vi "build.stepElement.parse.vi"(11 "steps in":variant[](array[variant])) -> (0 "error out":errorcluster, 3 "Flow Elements":T1[](array[typedef]))   [LabVIEW 2024]
uses:
  controls/UiStepBuilder.ctl
  controls/type.step-builder.ctl
  controls/typeStepVarients.ctl
  controls/type.StepFunction.ctl
  Polymorphics/variantCtrlString.vi
  Polymorphics/variantCtrlStepFunction.vi
  Polymorphics/variantCtrlSetpoint.vi
  Polymorphics/variantCtrlNumber.vi
  proc.util.validateParamExist.vi
  <vilib>/Utility/error.llb/Clear Errors.vi
  <vilib>/Utility/error.llb/Trim Whitespace One-Sided.vi
  util.error.create.vi
  Polymorphics/variantCtrlStepPointer.vi
  Polymorphics/variantCtrlStepProcPointer.vi
  Polymorphics/variantCtrlStepUserMessage.vi
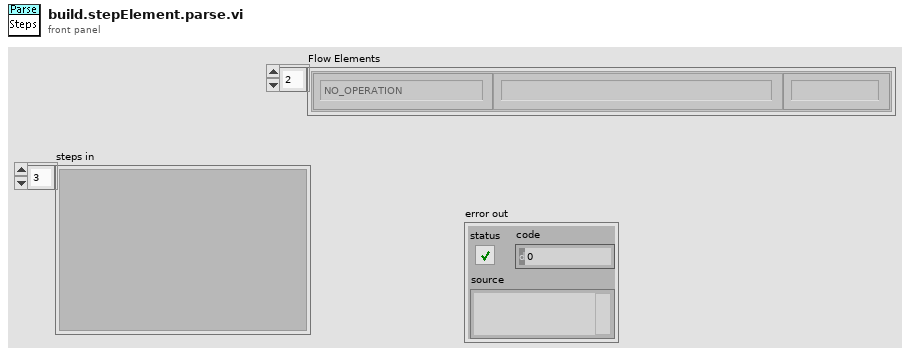
[diagram p1: front panel]
types:
  T1 = typedef "UiStepBuilder.ctl" = cluster{"Step Function":T2, "ParamString":string, "Step Label":string}
  T2 = typedef "type.step-builder.ctl" = enum16{"NO_OPERATION", "DELAY-JUMP", "DELAY", "JUMP", "COMPLETE", "SCHEDULER", "IRR-CHECK", "UNIT-CHECK", "UNIT-SAMPLE", "UNIT-DOSE", "LOG-REPORT", "LOG-MESSAGE", "IO-READ", "IO-READ-MANY", "IO-WRITE", "IO-COMPARE-OUT", "IO-COMPARE-IN", "PROC-START", "PROC-STOP", "PROC-LOAD", "PROC-IS-COMPLETED", "RECORD-MOVE", "GET-RH", "GET-UV", "GET-WD", "GET-WS", "OCS-CHECK", "OCS-RECORD"}
  T3 = typedef "typeStepVarients.ctl" = enum16{"stepNameID", "stepFunction", "stepReport", "stepSetpoint", "stepPointer", "stepProcPointer", "stepIoPointer", "stepIoValue", "stepFilePointer", "stepMessage", "stepTimeString", "stepNumReg", "stepStrReg", "stepSeconds", "stepUnitDoseParams", "stepUnitIndex"}
  T4 = typedef "type.StepFunction.ctl" = enum16{"__NO-OP", "_DELAY_LOAD", "_DELAY_COMPARE", "_JUMP", "_COMPLETE", "_COMPARE", "_LOG_MESSAGE", "_LOG_LAST_REPORT", "_SCHEDULE", "_SCHED_DAILY", "CLK_COMPARE", "PROC_START", "PROC_STOP", "PROC_LOAD", "PROC_COMPLETION_CHECK", "PROC_COMPLETION_LOAD", "_IO_READ", "_IO_READ_MANY", "_IO_WRITE", "_IO_WRITE_BY_REG", "_IO_GET_OUTPUT", "_OCS_CHECK", "_OCS_RECORD", "_GET_RH", "_GET_ACC_UV", "_GET_WD", "_GET_WS", "_REC_DELETE", "_REC_MOVE", "_REC_COPY", "_IRR_CHECK", "UNIT_CHECK", "UNIT_SAMPLE", "UNIT_DOSE"}
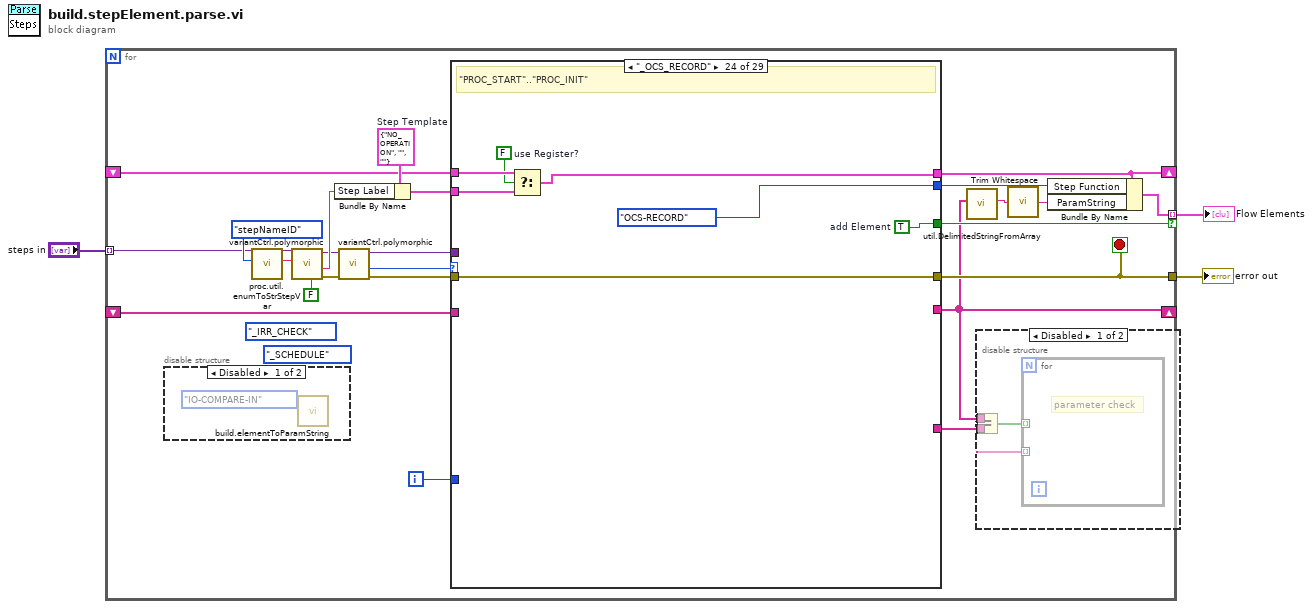
[diagram p0: block diagram]
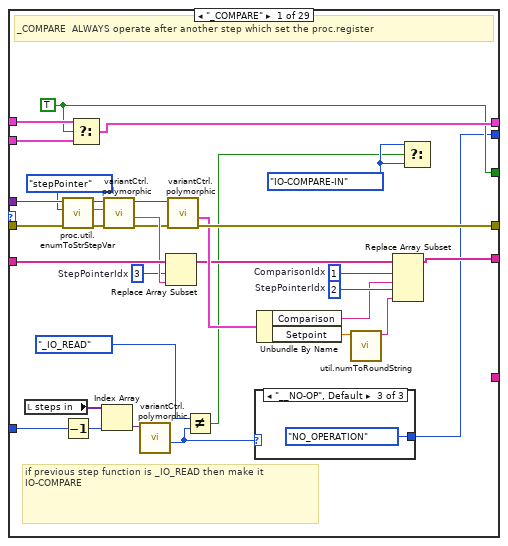
[diagram p4: hidden frame]
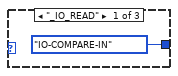
[diagram p5: hidden frame]
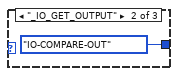
[diagram p6: hidden frame]
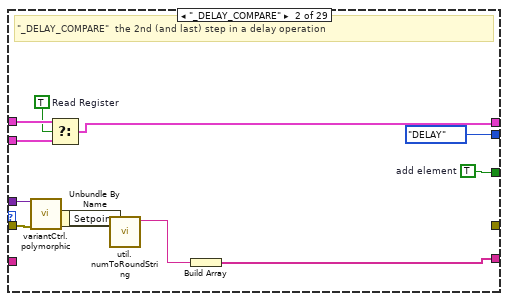
[diagram p7: hidden frame]
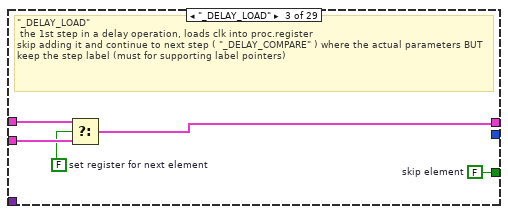
[diagram p8: hidden frame]
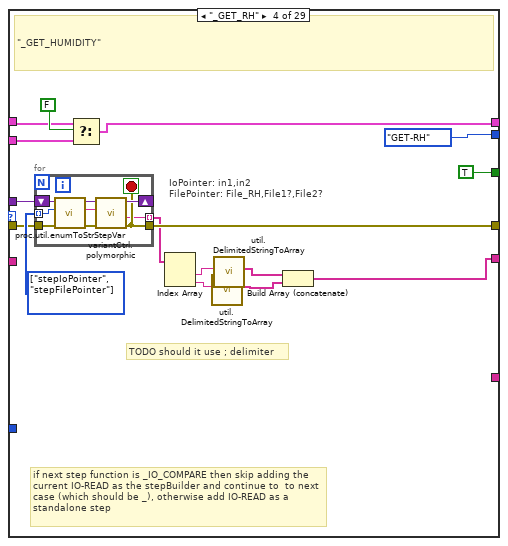
[diagram p9: hidden frame]
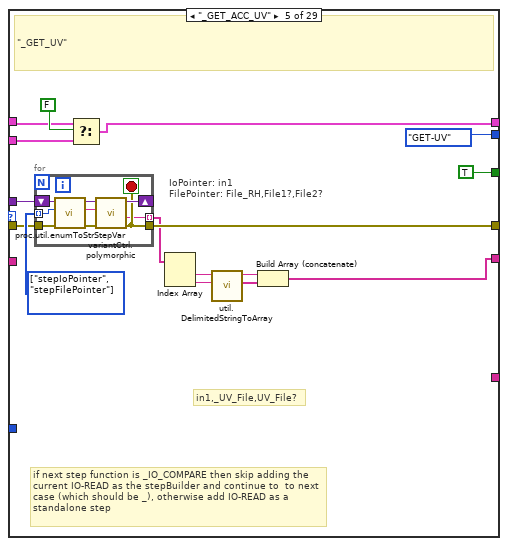
[diagram p10: hidden frame]
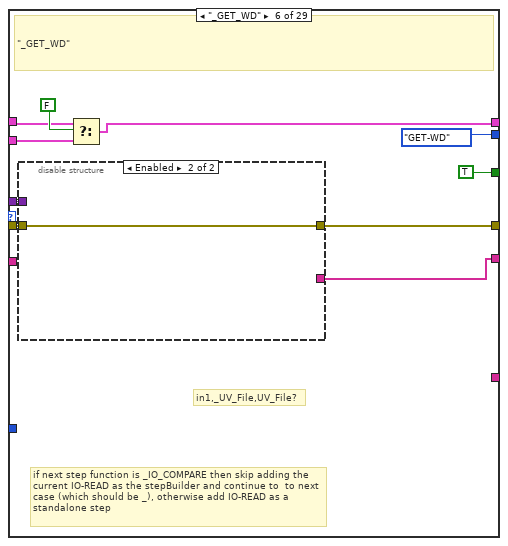
[diagram p11: hidden frame]
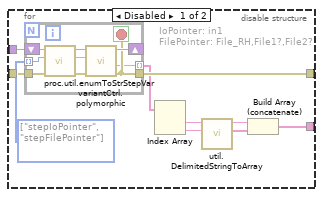
[diagram p12: hidden frame]
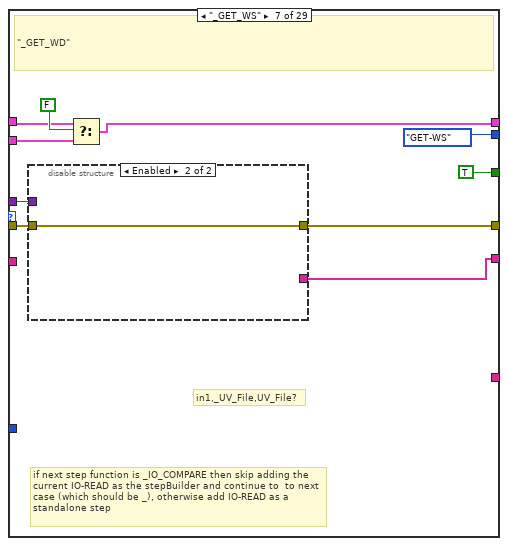
[diagram p13: hidden frame]
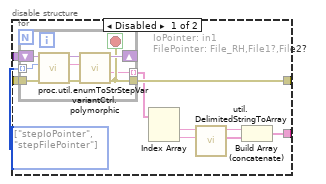
[diagram p14: hidden frame]
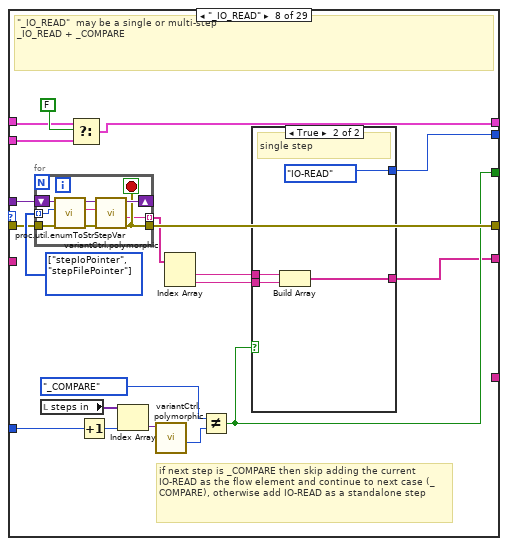
[diagram p15: hidden frame]
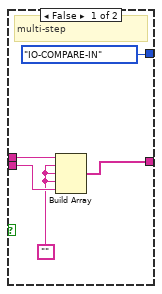
[diagram p16: hidden frame]
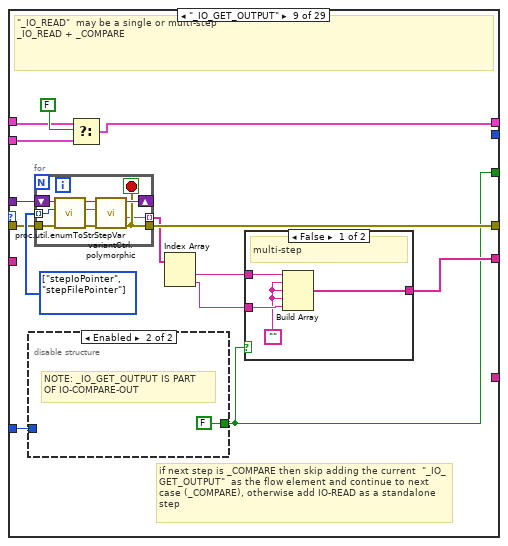
[diagram p17: hidden frame]
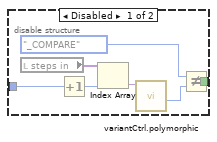
[diagram p18: hidden frame]
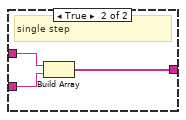
[diagram p19: hidden frame]
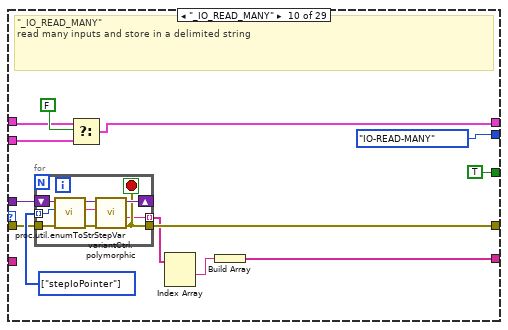
[diagram p20: hidden frame]
diagram:
  n1 = for {
    tunnel: "steps in" -> [w25] mode=indexing
    shift-right: [w9] -> _
    shift-left: _ -> [w18]
    tunnel: [w15] -> w2
    tunnel: [w10] -> w3 mode=indexing if=w14
    shift-right: [w5] -> _
    shift-left: _ -> [w13]
    i -> [w12]
    stop <- w15 stop-if-true
    (unwired) type.StepFunction."_SCHEDULE" ("StepFunction")
    (unwired) type.StepFunction."_IRR_CHECK" ("StepFunction")
    w22 = T1 {"Step Function"=enum."NO_OPERATION", "ParamString"="", "Step Label"=""}  # Step Template
    n2 = disable-structure shown="Disabled" {
      frame Disabled {
        n3 = call "build.elementToParamString.vi"("UiStepFunction"=type.step-builder."IO-COMPARE-IN") -> ()  [unwired: 9 in, 2 out]
      }
      frame Enabled {
      }
    }
    n4 = call "proc.util.enumToStrStepVar.vi"("Step var"=typeStepVarients."stepNameID") -> ("String"=w27:string)  [unwired: 10 in]
    n5 = call-poly "variantCtrl.polymorphic.vi"("isRequired (T)"=FALSE, "name in"=w27, "Step in"=w25) -> ("error out"=w20:errorcluster, "String Value"=w23:string, "Step out"=w21:variant)  [unwired: 5 in, 1 out]
    n6 = Bundle By Name(cluster=w22, "Step Label"=w23) -> (w19:T1)
    n7 = call-poly "variantCtrl.polymorphic.vi"("error in"=w20, "variant in"=w21) -> ("error out"=w16:errorcluster, "StepFunction"=w6:T4, "variant out"=w17:variant)  [unwired: 6 in, 1 out]
    n8 = case shown="\"_OCS_RECORD\"" w6 {
      selector: w6 -> [_ _ _ _ _ _ _ _ _ _ _ _ _ _ _ _ _ _ _ _ _ _ _ _ _ _ _ _ w507]
      tunnel: w19 -> [w61 w73 w80 w96 w118 w135 w162 w199 w229 w264 w283 w299 w307 w315 w327 w340 w353 w365 w384 w397 w410 w424 w432 w439 w452 w466 w480 w491 _]
      tunnel: [w60 w68 w81 w90 w112 w131 w158 w185 w220 w258 w278 w294 w303 w311 w324 w336 w349 w359 w379 w392 w405 w420 w428 w435 w448 w462 w476 w487 w503] -> w9
      tunnel: w18 -> [w62 w72 w82 w97 w119 w136 w163 w200 w230 w265 w284 w300 w308 w316 w328 w341 w354 w366 w385 w398 w411 w425 w433 w440 w453 w467 w481 w492 w503]
      tunnel: w17 -> [w59 w77 _ w95 w117 w134 w161 w198 w228 w263 w282 w302 _ w318 w330 w343 w348 w364 w387 w400 w413 w427 _ _ w455 w469 w483 w494 _]
      tunnel: w16 -> [w57 w75 _ w93 w115 w133 w160 w196 w226 w261 w280 w301 _ w317 w329 w342 w347 w362 w386 w399 w412 w426 w434 w441 w454 w468 w482 w493 _]
      tunnel: [w51 _ _ w92 w114 w132 w159 w195 w225 w260 w279 _ _ _ _ w335 w346 w361 w375 w388 w401 w418 w434 w441 w447 w461 w475 w486 w504] -> w15
      tunnel: [w35 w67 w79 TRUE ("s") TRUE ("s") TRUE ("s") TRUE ("s") w184 w218 TRUE ("add Element") TRUE ("s") w295 w304 w312 w325 w337 w350 TRUE ("s") w380 w393 w406 w421 w429 w436 w449 w463 w477 w488 _] -> w14
      tunnel: [w36 w66 _ w83 w107 w128 w155 w182 w219 w254 w275 w293 _ w310 w320 w331 w344 w355 w378 w391 w404 w419 _ _ w442 w456 w470 w485 _] -> w5
      tunnel: w13 -> [w55 _ _ _ _ _ _ _ _ _ _ _ _ _ w323 _ _ _ _ _ _ _ _ _ _ _ _ _ _]
      tunnel: w12 -> [w38 _ _ _ _ _ _ w190 w221 _ _ _ _ _ _ _ _ _ _ _ _ _ _ _ _ _ _ _ _]
      tunnel: [w32 type.step-builder."DELAY" ("UiStepFunction") _ type.step-builder."GET-RH" ("UiStepFunction") type.step-builder."GET-UV" ("UiStepFunction") type.step-builder."GET-WD" ("UiStepFunction") type.step-builder."GET-WS" ("UiStepFunction") w183 _ type.step-builder."IO-READ-MANY" ("UiStepFunction") type.step-builder."IO-WRITE" ("UiStepFunction") type.step-builder."JUMP" ("UiStepFunction") type.step-builder."COMPLETE" ("UiStepFunction") _ type.step-builder."PROC-IS-COMPLETED" ("UiStepFunction") type.step-builder."LOG-REPORT" ("UiStepFunction") type.step-builder."LOG-MESSAGE" ("UiStepFunction") type.step-builder."RECORD-MOVE" ("UiStepFunction") type.step-builder."PROC-START" ("UiStepFunction") type.step-builder."PROC-STOP" ("UiStepFunction") type.step-builder."PROC-LOAD" ("UiStepFunction") type.step-builder."IRR-CHECK" ("UiStepFunction") type.step-builder."OCS-CHECK" ("UiStepFunction") type.step-builder."OCS-RECORD" ("UiStepFunction") type.step-builder."UNIT-CHECK" ("UiStepFunction") type.step-builder."UNIT-SAMPLE" ("UiStepFunction") type.step-builder."UNIT-SAMPLE" ("UiStepFunction") type.step-builder."SCHEDULER" ("UiStepFunction") type.step-builder."NO_OPERATION" ("UiStepFunction")] -> w11
      tunnel: [_ _ _ _ _ _ _ _ _ _ string[] ["Out", "Value:Timeout", "File?"] ("params") _ _ _ _ _ _ _ _ _ _ _ _ _ _ _ _ _ _] -> w4
      frame "_COMPARE" {
        w46 = 1  # ComparisonIdx
        w47 = 2  # StepPointerIdx
        w53 = 3  # StepPointerIdx
        w37 = type.step-builder."IO-COMPARE-IN" ("UiStepFunction")
        w35 = TRUE ("s")
        # "if previous step function is _IO_READ then make it IO-COMPARE"
        # "_COMPARE  ALWAYS operate after another step which set the proc.register"
        n9 = local read "steps in"() -> (w42:variant[])
        n10 = call "proc.util.enumToStrStepVar.vi"("Step var"=typeStepVarients."stepPointer") -> ("String"=w56:string)  [unwired: 10 in]
        n11 = Decrement(x=w38) -> (x-1=w41:i32)
        n12 = Select(t=w62, s=w35, f=w61) -> (s? t:f=w60:T1)
        n13 = Index Array(array=w42, index=w41) -> (element=w40:variant)
        n14 = call-poly "variantCtrl.polymorphic.vi"("error in"=w57, "name in"=w56, "Step in"=w59) -> ("error out"=w50:errorcluster, "String Value"=w54:string, "Step out"=w52:variant)  [unwired: 5 in, 1 out]
        n15 = call-poly "variantCtrl.polymorphic.vi"("variant in"=w40) -> ("StepFunction"=w33:T4)  [unwired: 7 in, 3 out]
        n16 = Replace Array Subset(array=w55, new element=w54, index=w53) -> (w48:string[])
        n17 = call-poly "variantCtrl.polymorphic.vi"("error in"=w50, "procElement in in"=w52) -> ("error out"=w51:errorcluster, "setpoint"=w49:cluster{"Comparison":string, "Setpoint":dbl})  [unwired: 6 in, 2 out]
        n18 = Not Equal?(x=type.StepFunction."_IO_READ" ("StepFunction"), y=w33) -> (x != y?=w34:bool)
        n19 = case shown="\"__NO-OP\", Default" w33 {
          tunnel: [type.step-builder."IO-COMPARE-IN" ("UiStepFunction") type.step-builder."IO-COMPARE-OUT" ("UiStepFunction") type.step-builder."NO_OPERATION" ("UiStepFunction")] -> w32
          frame "_IO_READ" {
          }
          frame "_IO_GET_OUTPUT" {
          }
          frame "__NO-OP", Default {
          }
        }
        n20 = Unbundle By Name(w49) -> ("Comparison"=w45:string, "Setpoint"=w44:dbl)
        n21 = call "util.numToRoundString.vi"("reg in"=w44) -> ("String"=w43:string)  [unwired: 10 in]
        n22 = Replace Array Subset(array=w48, new element #1=w45, index #1=w46, new element #2=w43, index #2=w47) -> (w36:string[])
        n23 = Select(t=w37, s=w34, f=w37) -> ()  [unwired: 1 out]
      }
      frame "_DELAY_COMPARE" {
        w67 = TRUE  # add element
        w69 = TRUE  # Read Register
        # "\"_DELAY_COMPARE\"  the 2nd (and last) step in a delay operation"
        n24 = call-poly "variantCtrl.polymorphic.vi"("error in"=w75, "procElement in in"=w77) -> ("setpoint"=w76:cluster{"Comparison":string, "Setpoint":dbl})  [unwired: 6 in, 3 out]
        n25 = Select(t=w72, s=w69, f=w73) -> (s? t:f=w68:T1)
        n26 = Unbundle By Name(w76) -> ("Setpoint"=w74:dbl)
        n27 = call "util.numToRoundString.vi"("reg in"=w74) -> ("String"=w70:string)  [unwired: 10 in]
        n28 = Build Array(w70) -> (w66:string[])
      }
      frame "_DELAY_LOAD" {
        w79 = FALSE  # skip element
        w78 = FALSE  # set register for next element
        # "\"_DELAY_LOAD\" \n the 1st step in a delay operation, loads clk into proc.register\nskip adding it and continue to next step ( \"_DELAY_COMPARE\" ) where the actual parameters BUT keep the step label (must for supporting label pointers)"
        n29 = Select(t=w82, s=w78, f=w80) -> (s? t:f=w81:T1)
      }
      frame "_GET_RH" {
        w94 = T3[] [enum."stepIoPointer", enum."stepFilePointer"] items=["stepNameID", "stepFunction", "stepReport", "stepSetpoint", "stepPointer", "stepProcPointer", "stepIoPointer", "stepIoValue", "stepFilePointer", "stepMessage", "stepTimeString", "stepNumReg", "stepStrReg", "stepSeconds", "stepUnitDoseParams", "stepUnitIndex"] ("Step var")
        # "TODO should it use ; delimiter"
        # "IoPointer: in1,in2\nFilePointer: File_RH,File1?,File2?"
        # "if next step function is _IO_COMPARE then skip adding the current IO-READ as the stepBuilder and continue to  to next case (which should be _), otherwise add IO-READ as a standalone step"
        # "\"_GET_HUMIDITY\""
        n30 = for {
          tunnel: w94 -> [w103] mode=indexing
          shift-right: [w101] -> _
          shift-left: w95 -> [w104]
          tunnel: w93 -> [w105]
          tunnel: [w100] -> w92
          tunnel: [w99] -> w91 mode=indexing
          stop <- w100 stop-if-true
          n31 = call "proc.util.enumToStrStepVar.vi"("Step var"=w103) -> ("String"=w102:string)  [unwired: 10 in]
          n32 = call-poly "variantCtrl.polymorphic.vi"("error in"=w105, "name in"=w102, "Step in"=w104) -> ("error out"=w100:errorcluster, "String Value"=w99:string, "Step out"=w101:variant)  [unwired: 5 in, 1 out]
        }
        n33 = Select(t=w97, s=FALSE, f=w96) -> (s? t:f=w90:T1)
        n34 = Index Array(array=w91) -> (element #1=w88:string, element #2=w86:string)  [unwired: 2 in]
        n35 = call "util.DelimitedStringToArray.vi"("delimitaed string"=w86) -> ("array out"=w85:string[])  [unwired: 10 in]
        n36 = call "util.DelimitedStringToArray.vi"("delimitaed string"=w88) -> ("array out"=w87:string[])  [unwired: 10 in]
        n37 = Build Array (concatenate)(w87, w85) -> (w83:string[])
      }
      frame "_GET_ACC_UV" {
        w116 = T3[] [enum."stepIoPointer", enum."stepFilePointer"] items=["stepNameID", "stepFunction", "stepReport", "stepSetpoint", "stepPointer", "stepProcPointer", "stepIoPointer", "stepIoValue", "stepFilePointer", "stepMessage", "stepTimeString", "stepNumReg", "stepStrReg", "stepSeconds", "stepUnitDoseParams", "stepUnitIndex"] ("Step var")
        # "in1,_UV_File,UV_File?"
        # "IoPointer: in1\nFilePointer: File_RH,File1?,File2?"
        # "if next step function is _IO_COMPARE then skip adding the current IO-READ as the stepBuilder and continue to  to next case (which should be _), otherwise add IO-READ as a standalone step"
        # "\"_GET_UV\""
        n38 = for {
          tunnel: w116 -> [w125] mode=indexing
          shift-right: [w123] -> _
          shift-left: w117 -> [w126]
          tunnel: w115 -> [w127]
          tunnel: [w122] -> w114
          tunnel: [w121] -> w113 mode=indexing
          stop <- w122 stop-if-true
          n39 = call "proc.util.enumToStrStepVar.vi"("Step var"=w125) -> ("String"=w124:string)  [unwired: 10 in]
          n40 = call-poly "variantCtrl.polymorphic.vi"("error in"=w127, "name in"=w124, "Step in"=w126) -> ("error out"=w122:errorcluster, "String Value"=w121:string, "Step out"=w123:variant)  [unwired: 5 in, 1 out]
        }
        n41 = Select(t=w119, s=FALSE, f=w118) -> (s? t:f=w112:T1)
        n42 = Index Array(array=w113) -> (element #1=w106:string, element #2=w110:string)  [unwired: 2 in]
        n43 = call "util.DelimitedStringToArray.vi"("delimitaed string"=w110) -> ("array out"=w109:string[])  [unwired: 10 in]
        n44 = Build Array (concatenate)(w106, w109) -> (w107:string[])
      }
      frame "_GET_WD" {
        # "in1,_UV_File,UV_File?"
        # "if next step function is _IO_COMPARE then skip adding the current IO-READ as the stepBuilder and continue to  to next case (which should be _), otherwise add IO-READ as a standalone step"
        # "\"_GET_WD\""
        n45 = disable-structure shown="Enabled" {
          disable-tunnel: w134 -> [w146 _]
          disable-tunnel: w133 -> [w144 w154]
          disable-tunnel: [w143 w154] -> w132
          disable-tunnel: [w139 _] -> w128
          frame Disabled {
            w145 = T3[] [enum."stepIoPointer", enum."stepFilePointer"] items=["stepNameID", "stepFunction", "stepReport", "stepSetpoint", "stepPointer", "stepProcPointer", "stepIoPointer", "stepIoValue", "stepFilePointer", "stepMessage", "stepTimeString", "stepNumReg", "stepStrReg", "stepSeconds", "stepUnitDoseParams", "stepUnitIndex"] ("Step var")
            # "IoPointer: in1\nFilePointer: File_RH,File1?,File2?"
            n46 = for {
              tunnel: w145 -> [w151] mode=indexing
              shift-right: [w149] -> _
              shift-left: w146 -> [w152]
              tunnel: w144 -> [w153]
              tunnel: [w148] -> w143
              tunnel: [w147] -> w142 mode=indexing
              stop <- w148 stop-if-true
              n47 = call "proc.util.enumToStrStepVar.vi"("Step var"=w151) -> ("String"=w150:string)  [unwired: 10 in]
              n48 = call-poly "variantCtrl.polymorphic.vi"("error in"=w153, "name in"=w150, "Step in"=w152) -> ("error out"=w148:errorcluster, "String Value"=w147:string, "Step out"=w149:variant)  [unwired: 5 in, 1 out]
            }
            n49 = Index Array(array=w142) -> (element #1=w138:string, element #2=w141:string)  [unwired: 2 in]
            n50 = call "util.DelimitedStringToArray.vi"("delimitaed string"=w141) -> ("array out"=w140:string[])  [unwired: 10 in]
            n51 = Build Array (concatenate)(w138, w140) -> (w139:string[])
          }
          frame Enabled {
          }
        }
        n52 = Select(t=w136, s=FALSE, f=w135) -> (s? t:f=w131:T1)
      }
      frame "_GET_WS" {
        # "in1,_UV_File,UV_File?"
        # "if next step function is _IO_COMPARE then skip adding the current IO-READ as the stepBuilder and continue to  to next case (which should be _), otherwise add IO-READ as a standalone step"
        # "\"_GET_WD\""
        n53 = disable-structure shown="Enabled" {
          disable-tunnel: w161 -> [w173 _]
          disable-tunnel: w160 -> [w171 w181]
          disable-tunnel: [w170 w181] -> w159
          disable-tunnel: [w166 _] -> w155
          frame Disabled {
            w172 = T3[] [enum."stepIoPointer", enum."stepFilePointer"] items=["stepNameID", "stepFunction", "stepReport", "stepSetpoint", "stepPointer", "stepProcPointer", "stepIoPointer", "stepIoValue", "stepFilePointer", "stepMessage", "stepTimeString", "stepNumReg", "stepStrReg", "stepSeconds", "stepUnitDoseParams", "stepUnitIndex"] ("Step var")
            # "IoPointer: in1\nFilePointer: File_RH,File1?,File2?"
            n54 = for {
              tunnel: w172 -> [w178] mode=indexing
              shift-right: [w176] -> _
              shift-left: w173 -> [w179]
              tunnel: w171 -> [w180]
              tunnel: [w175] -> w170
              tunnel: [w174] -> w169 mode=indexing
              stop <- w175 stop-if-true
              n55 = call "proc.util.enumToStrStepVar.vi"("Step var"=w178) -> ("String"=w177:string)  [unwired: 10 in]
              n56 = call-poly "variantCtrl.polymorphic.vi"("error in"=w180, "name in"=w177, "Step in"=w179) -> ("error out"=w175:errorcluster, "String Value"=w174:string, "Step out"=w176:variant)  [unwired: 5 in, 1 out]
            }
            n57 = Index Array(array=w169) -> (element #1=w165:string, element #2=w168:string)  [unwired: 2 in]
            n58 = call "util.DelimitedStringToArray.vi"("delimitaed string"=w168) -> ("array out"=w167:string[])  [unwired: 10 in]
            n59 = Build Array (concatenate)(w165, w167) -> (w166:string[])
          }
          frame Enabled {
          }
        }
        n60 = Select(t=w163, s=FALSE, f=w162) -> (s? t:f=w158:T1)
      }
      frame "_IO_READ" {
        w197 = T3[] [enum."stepIoPointer", enum."stepFilePointer"] items=["stepNameID", "stepFunction", "stepReport", "stepSetpoint", "stepPointer", "stepProcPointer", "stepIoPointer", "stepIoValue", "stepFilePointer", "stepMessage", "stepTimeString", "stepNumReg", "stepStrReg", "stepSeconds", "stepUnitDoseParams", "stepUnitIndex"] ("Step var")
        # "if next step is _COMPARE then skip adding the current IO-READ as the flow element and continue to next case (_COMPARE), otherwise add IO-READ as a standalone step"
        # "\"_IO_READ\"  may be a single or multi-step\n_IO_READ + _COMPARE"
        n61 = for {
          tunnel: w197 -> [w215] mode=indexing
          shift-right: [w213] -> _
          shift-left: w198 -> [w216]
          tunnel: w196 -> [w217]
          tunnel: [w212] -> w195
          tunnel: [w211] -> w194 mode=indexing
          stop <- w212 stop-if-true
          n62 = call "proc.util.enumToStrStepVar.vi"("Step var"=w215) -> ("String"=w214:string)  [unwired: 10 in]
          n63 = call-poly "variantCtrl.polymorphic.vi"("error in"=w217, "name in"=w214, "Step in"=w216) -> ("error out"=w212:errorcluster, "String Value"=w211:string, "Step out"=w213:variant)  [unwired: 5 in, 1 out]
        }
        n64 = local read "steps in"() -> (w191:variant[])
        n65 = Select(t=w200, s=FALSE, f=w199) -> (s? t:f=w185:T1)
        n66 = Increment(x=w190) -> (x+1=w189:i32)
        n67 = Index Array(array=w191, index=w189) -> (element=w188:variant)
        n68 = call-poly "variantCtrl.polymorphic.vi"("variant in"=w188) -> ("StepFunction"=w186:T4)  [unwired: 7 in, 3 out]
        n69 = Index Array(array=w194) -> (element #1=w193:string, element #2=w192:string)  [unwired: 2 in]
        n70 = Not Equal?(x=type.StepFunction."_COMPARE" ("StepFunction"), y=w186) -> (x != y?=w184:bool)
        n71 = case shown="True" w184 {
          tunnel: w193 -> [w206 w210]
          tunnel: w192 -> [w205 w208]
          tunnel: [w203 w209] -> w182
          tunnel: [type.step-builder."IO-COMPARE-IN" ("UiStepFunction") type.step-builder."IO-READ" ("UiStepFunction")] -> w183
          frame False {
            w204 = ""
            # "multi-step"
            n72 = Build Array(w206, w204, w204, w204, w205) -> (w203:string[])
          }
          frame True {
            # "single step"
            n73 = Build Array(w210, w208) -> (w209:string[])
          }
        }
      }
      frame "_IO_GET_OUTPUT" {
        w227 = T3[] [enum."stepIoPointer", enum."stepFilePointer"] items=["stepNameID", "stepFunction", "stepReport", "stepSetpoint", "stepPointer", "stepProcPointer", "stepIoPointer", "stepIoValue", "stepFilePointer", "stepMessage", "stepTimeString", "stepNumReg", "stepStrReg", "stepSeconds", "stepUnitDoseParams", "stepUnitIndex"] ("Step var")
        # "if next step is _COMPARE then skip adding the current  \"_IO_GET_OUTPUT\"  as the flow element and continue to next case (_COMPARE), otherwise add IO-READ as a standalone step"
        # "\"_IO_READ\"  may be a single or multi-step\n_IO_READ + _COMPARE"
        n74 = disable-structure shown="Enabled" {
          disable-tunnel: w221 -> [w237 _]
          disable-tunnel: [w232 FALSE] -> w218
          frame Disabled {
            n75 = local read "steps in"() -> (w238:variant[])
            n76 = Increment(x=w237) -> (x+1=w236:i32)
            n77 = Index Array(array=w238, index=w236) -> (element=w235:variant)
            n78 = call-poly "variantCtrl.polymorphic.vi"("variant in"=w235) -> ("StepFunction"=w233:T4)  [unwired: 7 in, 3 out]
            n79 = Not Equal?(x=type.StepFunction."_COMPARE" ("StepFunction"), y=w233) -> (x != y?=w232:bool)
          }
          frame Enabled {
            # "NOTE: _IO_GET_OUTPUT IS PART\nOF IO-COMPARE-OUT"
          }
        }
        n80 = for {
          tunnel: w227 -> [w251] mode=indexing
          shift-right: [w249] -> _
          shift-left: w228 -> [w252]
          tunnel: w226 -> [w253]
          tunnel: [w248] -> w225
          tunnel: [w247] -> w224 mode=indexing
          stop <- w248 stop-if-true
          n81 = call "proc.util.enumToStrStepVar.vi"("Step var"=w251) -> ("String"=w250:string)  [unwired: 10 in]
          n82 = call-poly "variantCtrl.polymorphic.vi"("error in"=w253, "name in"=w250, "Step in"=w252) -> ("error out"=w248:errorcluster, "String Value"=w247:string, "Step out"=w249:variant)  [unwired: 5 in, 1 out]
        }
        n83 = Select(t=w230, s=FALSE, f=w229) -> (s? t:f=w220:T1)
        n84 = Index Array(array=w224) -> (element #1=w223:string, element #2=w222:string)  [unwired: 2 in]
        n85 = case shown="False" w218 {
          tunnel: w223 -> [w243 w246]
          tunnel: w222 -> [w242 w244]
          tunnel: [w240 w245] -> w219
          frame False {
            w241 = ""
            # "multi-step"
            n86 = Build Array(w243, w241, w241, w241, w242) -> (w240:string[])
          }
          frame True {
            # "single step"
            n87 = Build Array(w246, w244) -> (w245:string[])
          }
        }
      }
      frame "_IO_READ_MANY" {
        w262 = T3[] [enum."stepIoPointer"] items=["stepNameID", "stepFunction", "stepReport", "stepSetpoint", "stepPointer", "stepProcPointer", "stepIoPointer", "stepIoValue", "stepFilePointer", "stepMessage", "stepTimeString", "stepNumReg", "stepStrReg", "stepSeconds", "stepUnitDoseParams", "stepUnitIndex"] ("Step var")
        # "\"_IO_READ_MANY\" \nread many inputs and store in a delimited string"
        n88 = for {
          tunnel: w262 -> [w271] mode=indexing
          shift-right: [w269] -> _
          shift-left: w263 -> [w272]
          tunnel: w261 -> [w273]
          tunnel: [w268] -> w260
          tunnel: [w267] -> w259 mode=indexing
          stop <- w268 stop-if-true
          n89 = call "proc.util.enumToStrStepVar.vi"("Step var"=w271) -> ("String"=w270:string)  [unwired: 10 in]
          n90 = call-poly "variantCtrl.polymorphic.vi"("error in"=w273, "name in"=w270, "Step in"=w272) -> ("error out"=w268:errorcluster, "String Value"=w267:string, "Step out"=w269:variant)  [unwired: 5 in, 1 out]
        }
        n91 = Select(t=w265, s=FALSE, f=w264) -> (s? t:f=w258:T1)
        n92 = Index Array(array=w259) -> (element #1=w255:string)  [unwired: 2 in, 1 out]
        n93 = Build Array(w255) -> (w254:string[])
      }
      frame "_IO_WRITE" {
        w281 = T3[] [enum."stepIoPointer", enum."stepIoValue", enum."stepFilePointer"] items=["stepNameID", "stepFunction", "stepReport", "stepSetpoint", "stepPointer", "stepProcPointer", "stepIoPointer", "stepIoValue", "stepFilePointer", "stepMessage", "stepTimeString", "stepNumReg", "stepStrReg", "stepSeconds", "stepUnitDoseParams", "stepUnitIndex"] ("Step var")
        # "\"_IO_WRITE\""
        n94 = for {
          tunnel: w281 -> [w290] mode=indexing
          shift-right: [w288] -> _
          shift-left: w282 -> [w291]
          tunnel: w280 -> [w292]
          tunnel: [w287] -> w279
          tunnel: [w286] -> w275 mode=indexing
          stop <- w287 stop-if-true
          n95 = call "proc.util.enumToStrStepVar.vi"("Step var"=w290) -> ("String"=w289:string)  [unwired: 10 in]
          n96 = call-poly "variantCtrl.polymorphic.vi"("error in"=w292, "name in"=w289, "Step in"=w291) -> ("error out"=w287:errorcluster, "String Value"=w286:string, "Step out"=w288:variant)  [unwired: 5 in, 1 out]
        }
        n97 = Select(t=w284, s=FALSE, f=w283) -> (s? t:f=w278:T1)
      }
      frame "_JUMP" {
        w295 = TRUE  # add Element
        w296 = FALSE  # Read Register?
        # "\"_JUMP\"  single step"
        n98 = call-poly "variantCtrl.polymorphic.vi"("error in"=w301, "stepElement in in"=w302) -> ("string out"=w297:string)  [unwired: 6 in, 3 out]
        n99 = Select(t=w300, s=w296, f=w299) -> (s? t:f=w294:T1)
        n100 = Build Array(w297) -> (w293:string[])
      }
      frame "_COMPLETE" {
        w304 = TRUE  # add Element
        w305 = FALSE  # Read Register?
        # "\"_COMPLETE\""
        n101 = Select(t=w308, s=w305, f=w307) -> (s? t:f=w303:T1)
      }
      frame "PROC_COMPLETION_LOAD" {
        w312 = FALSE  # skip Element
        w313 = FALSE  # Read Register?
        # "\"_JUMP\"  single step"
        n102 = call-poly "variantCtrl.polymorphic.vi"("error in"=w317, "stepElement in in"=w318) -> ("string out"=w314:string)  [unwired: 6 in, 3 out]
        n103 = Select(t=w316, s=w313, f=w315) -> (s? t:f=w311:T1)
        n104 = Build Array "Build Param Array"(w314, "") -> (w310:string[])
      }
      frame "PROC_COMPLETION_CHECK" {
        w321 = 1  # StepPointer
        w325 = TRUE  # add Element
        w326 = TRUE  # Read Register?
        # "\"_JUMP\"  single step"
        n105 = call-poly "variantCtrl.polymorphic.vi"("error in"=w329, "stepElement in in"=w330) -> ("string out"=w322:string)  [unwired: 6 in, 3 out]
        n106 = Select(t=w328, s=w326, f=w327) -> (s? t:f=w324:T1)
        n107 = Replace Array Subset(array=w323, new element=w322, index=w321) -> (w320:string[])
      }
      frame "_LOG_LAST_REPORT" {
        w337 = TRUE  # add element
        # "\"_LOG_LAST_REPORT\"  single step"
        n108 = call "proc.util.enumToStrStepVar.vi"("Step var"=typeStepVarients."stepFilePointer" ("step variants")) -> ("String"=w334:string)  [unwired: 10 in]
        n109 = Select(t=w341, s=FALSE, f=w340) -> (s? t:f=w336:T1)
        n110 = call-poly "variantCtrl.polymorphic.vi"("error in"=w342, "name in"=w334, "Step in"=w343) -> ("error out"=w335:errorcluster, "String Value"=w332:string)  [unwired: 5 in, 2 out]
        n111 = Build Array(w332) -> (w331:string[])
      }
      frame "_LOG_MESSAGE" {
        w350 = TRUE  # add Step
        # "\"_LOG_MESSAGE\"  single step"
        n112 = Select(t=w354, s=FALSE, f=w353) -> (s? t:f=w349:T1)
        n113 = call-poly "variantCtrl.polymorphic.vi"("error in"=w347, "stepElement in in"=w348) -> ("error out"=w346:errorcluster, "string out"=w345:string)  [unwired: 6 in, 2 out]
        n114 = Build Array(w345) -> (w344:string[])
      }
      frame "_REC_MOVE" {
        w363 = T3[] [enum."stepFilePointer"] items=["stepNameID", "stepFunction", "stepReport", "stepSetpoint", "stepPointer", "stepProcPointer", "stepIoPointer", "stepIoValue", "stepFilePointer", "stepMessage", "stepTimeString", "stepNumReg", "stepStrReg", "stepSeconds", "stepUnitDoseParams", "stepUnitIndex"] ("Step var")
        # "IoPointer: in1,in2\nFilePointer: File_RH,File1?,File2?"
        # "if next step function is _IO_COMPARE then skip adding the current IO-READ as the stepBuilder and continue to  to next case (which should be _), otherwise add IO-READ as a standalone step"
        # "\"_RECORD_FILE_MOVE\" \n\n(1) source file\n(2) destination file"
        n115 = for {
          tunnel: w363 -> [w372] mode=indexing
          shift-right: [w370] -> _
          shift-left: w364 -> [w373]
          tunnel: w362 -> [w374]
          tunnel: [w369] -> w361
          tunnel: [w368] -> w360 mode=indexing
          stop <- w369 stop-if-true
          n116 = call "proc.util.enumToStrStepVar.vi"("Step var"=w372) -> ("String"=w371:string)  [unwired: 10 in]
          n117 = call-poly "variantCtrl.polymorphic.vi"("error in"=w374, "name in"=w371, "Step in"=w373) -> ("error out"=w369:errorcluster, "String Value"=w368:string, "Step out"=w370:variant)  [unwired: 5 in, 1 out]
        }
        n118 = Select(t=w366, s=FALSE, f=w365) -> (s? t:f=w359:T1)
        n119 = Index Array(array=w360) -> (element=w357:string)  [unwired: 1 in]
        n120 = call "util.DelimitedStringToArray.vi"("delimitaed string"=w357) -> ("array out"=w355:string[])  [unwired: 10 in]
      }
      frame "PROC_START" {
        w380 = TRUE  # add Element
        w381 = FALSE  # use Register?
        # "\"PROC_START\"..\"PROC_INIT\""
        n121 = Select(t=w385, s=w381, f=w384) -> (s? t:f=w379:T1)
        n122 = call "proc.util.enumToStrStepVar.vi"("Step var"=typeStepVarients."stepProcPointer") -> ("String"=w376:string)  [unwired: 10 in]
        n123 = call-poly "variantCtrl.polymorphic.vi"("error in"=w386, "name in"=w376, "Step in"=w387) -> ("error out"=w375:errorcluster, "String Value"=w382:string)  [unwired: 5 in, 2 out]
        n124 = Build Array(w382) -> (w378:string[])
      }
      frame "PROC_STOP" {
        w393 = TRUE  # add Element
        w394 = FALSE  # use Register?
        n125 = Select(t=w398, s=w394, f=w397) -> (s? t:f=w392:T1)
        n126 = call "proc.util.enumToStrStepVar.vi"("Step var"=typeStepVarients."stepProcPointer") -> ("String"=w389:string)  [unwired: 10 in]
        n127 = call-poly "variantCtrl.polymorphic.vi"("error in"=w399, "name in"=w389, "Step in"=w400) -> ("error out"=w388:errorcluster, "String Value"=w395:string)  [unwired: 5 in, 2 out]
        n128 = Build Array(w395) -> (w391:string[])
      }
      frame "PROC_LOAD" {
        w406 = TRUE  # add Element
        w407 = FALSE  # use Register?
        # "\"PROC_START\"..\"PROC_INIT\""
        n129 = Select(t=w411, s=w407, f=w410) -> (s? t:f=w405:T1)
        n130 = call "proc.util.enumToStrStepVar.vi"("Step var"=typeStepVarients."stepProcPointer") -> ("String"=w402:string)  [unwired: 10 in]
        n131 = call-poly "variantCtrl.polymorphic.vi"("error in"=w412, "name in"=w402, "Step in"=w413) -> ("error out"=w401:errorcluster, "String Value"=w408:string)  [unwired: 5 in, 2 out]
        n132 = Build Array(w408) -> (w404:string[])
      }
      frame "_IRR_CHECK" {
        w421 = TRUE  # add Element
        w422 = FALSE  # use Register?
        # "\"PROC_START\"..\"PROC_INIT\""
        n133 = Select(t=w425, s=w422, f=w424) -> (s? t:f=w420:T1)
        n134 = call "proc.util.enumToStrStepVar.vi"("Step var"=typeStepVarients."stepSeconds") -> ("String"=w416:string)  [unwired: 10 in]
        n135 = call-poly "variantCtrl.polymorphic.vi"("error in"=w426, "name in"=w416, "variant in"=w427) -> ("error out"=w418:errorcluster, "number"=w415:dbl)  [unwired: 5 in, 2 out]
        n136 = Number To Decimal String(number=w415) -> (decimal integer string=w414:string)  [unwired: 1 in]
        n137 = Build Array(w414) -> (w419:string[])
      }
      frame "_OCS_CHECK" {
        w429 = TRUE  # add Element
        w430 = FALSE  # use Register?
        # "\"PROC_START\"..\"PROC_INIT\""
        n138 = Select(t=w433, s=w430, f=w432) -> (s? t:f=w428:T1)
      }
      frame "_OCS_RECORD" {
        w436 = TRUE  # add Element
        w437 = FALSE  # use Register?
        # "\"PROC_START\"..\"PROC_INIT\""
        n139 = Select(t=w440, s=w437, f=w439) -> (s? t:f=w435:T1)
      }
      frame "UNIT_CHECK" {
        w449 = TRUE  # add Element
        w450 = FALSE  # use Register?
        # "\"UNIT_CHECK\""
        n140 = Select(t=w453, s=w450, f=w452) -> (s? t:f=w448:T1)
        n141 = call "proc.util.enumToStrStepVar.vi"("Step var"=typeStepVarients."stepUnitIndex") -> ("String"=w445:string)  [unwired: 10 in]
        n142 = call-poly "variantCtrl.polymorphic.vi"("error in"=w454, "name in"=w445, "variant in"=w455) -> ("error out"=w447:errorcluster, "number"=w444:dbl)  [unwired: 5 in, 2 out]
        n143 = Number To Decimal String(number=w444) -> (decimal integer string=w443:string)  [unwired: 1 in]
        n144 = Build Array(w443) -> (w442:string[])
      }
      frame "UNIT_SAMPLE" {
        w463 = TRUE  # add Element
        w464 = FALSE  # use Register?
        # "\"UNIT_SAMPLE\""
        n145 = Select(t=w467, s=w464, f=w466) -> (s? t:f=w462:T1)
        n146 = call "proc.util.enumToStrStepVar.vi"("Step var"=typeStepVarients."stepUnitIndex") -> ("String"=w459:string)  [unwired: 10 in]
        n147 = call-poly "variantCtrl.polymorphic.vi"("error in"=w468, "name in"=w459, "variant in"=w469) -> ("error out"=w461:errorcluster, "number"=w458:dbl)  [unwired: 5 in, 2 out]
        n148 = Number To Decimal String(number=w458) -> (decimal integer string=w457:string)  [unwired: 1 in]
        n149 = Build Array(w457) -> (w456:string[])
      }
      frame "UNIT_DOSE" {
        w477 = TRUE  # add Element
        w478 = FALSE  # use Register?
        # "\"UNIT_DOSE\""
        n150 = Select(t=w481, s=w478, f=w480) -> (s? t:f=w476:T1)
        n151 = call "proc.util.enumToStrStepVar.vi"("Step var"=typeStepVarients."stepUnitIndex") -> ("String"=w473:string)  [unwired: 10 in]
        n152 = call-poly "variantCtrl.polymorphic.vi"("error in"=w482, "name in"=w473, "variant in"=w483) -> ("error out"=w475:errorcluster, "number"=w472:dbl)  [unwired: 5 in, 2 out]
        n153 = Number To Decimal String(number=w472) -> (decimal integer string=w471:string)  [unwired: 1 in]
        n154 = Build Array(w471) -> (w470:string[])
      }
      frame "_SCHEDULE" {
        w488 = TRUE  # add Element
        w489 = FALSE  # use Register?
        # "\"_SCHEDULE\""
        n155 = disable-structure shown="Enabled" {
          disable-tunnel: w494 -> [w500 _]
          disable-tunnel: w493 -> [w499 w501]
          disable-tunnel: [w498 w501] -> w486
          disable-tunnel: [w495 _] -> w484
          frame Enabled {
            n156 = call "proc.util.enumToStrStepVar.vi"("Step var"=typeStepVarients."stepStrReg") -> ("String"=w496:string)  [unwired: 10 in]
            n157 = call-poly "variantCtrl.polymorphic.vi"("error in"=w499, "name in"=w496, "Step in"=w500) -> ("error out"=w498:errorcluster, "String Value"=w495:string)  [unwired: 5 in, 2 out]
          }
          frame Disabled {
          }
        }
        n158 = Select(t=w492, s=w489, f=w491) -> (s? t:f=w487:T1)
        n159 = Build Array(w484) -> (w485:string[])
      }
      frame Default {
        n160 = Format Into String(format string="%s is undefind" ("source"), w507) -> (resulting string=w505:string)  [unwired: 2 in, 1 out]
        n161 = disable-structure shown="Enabled" {
          disable-tunnel: w505 -> [w509 _]
          disable-tunnel: [w508 _] -> w504
          frame Disabled {
            w510 = errorcluster {"status"=TRUE, "code"=-1, "source"=""}  # error (-1)
            n162 = Bundle By Name(cluster=w510, "source"=w509) -> (w508:errorcluster)
          }
          frame Enabled {
          }
        }
      }
    }
    n163 = call "util.DelimitedStringFromArray.vi"("params array in"=w5) -> ("delimited string out"=w7:string)  [unwired: 10 in]
    n164 = disable-structure shown="Disabled" {
      disable-tunnel: w5 -> [w30 _]
      disable-tunnel: w4 -> [w28 _]
      frame Disabled {
        n165 = Equal?(x=w30, y=w28) -> (x = y?=w29:bool[])
        n166 = for {
          tunnel: w29 -> [_] mode=indexing
          tunnel: w28 -> [_] mode=indexing
          # "parameter check"
        }
      }
      frame Enabled {
      }
    }
    n167 = call <vilib>:"Trim Whitespace.vi"("string"=w7) -> ("trimmed string"=w8:string)  [unwired: 1 in]
    n168 = Bundle By Name(cluster=w9, "Step Function"=w11, "ParamString"=w8) -> (w10:T1)
  }
  "Flow Elements" <- w3
  "error out" <- w2
